vi "MGCC_EnergyMgmt_EMS_HTB.vi"() -> ()   [LabVIEW 2016]
doc: "This VI implements two linear programming models for energy management. The VI uses load and PV forecasting results from the respective functions to generate dispatch of PV and battery for the next 24 hours. Other constraints on the battery and electricity price information are custom inputs and should be specified prior to executing this function."
uses:
  Communication/Global communication.vi
  Communication/Global communication output.vi
  <vilib>/imath/engines/lvmath2/RunTimeEngine/RangeToken/NIMS_Range_R2 - Integer.vi
  <instcachedir>/0/NIMS_Range_R2 - Integer_89B873E74E6E489885E44F751DD9C6BF.lvgen/NIMS_Range_R2 - Integer_89B873E74E6E489885E44F751DD9C6BF_000.vi
  <vilib>/imath/engines/lvmath2/RunTimeEngine/CommandStatement/MC_CommandStatement_break.vi
  <vilib>/imath/engines/lvmath2/RunTimeEngine/VariableToken/NIMS_VariableToken_CondDefinedDefinedByReplace.vi
  <instcachedir>/0/NIMS_VariableToken_CondDefinedDefinedByReplace_D162CFFC24174562A9FEA619A91E1A56.lvgen/NIMS_VariableToken_CondDefinedDefinedByReplace_D162CFFC24174562A9FEA619A91E1A56_004.vi
  <vilib>/imath/engines/lvmath2/RunTimeEngine/IndexRead/NIMS V(R2).vi
  <instcachedir>/0/NIMS V(R2)_C76619605A0E4E9F8B2FA9389712AC47.lvgen/NIMS V(R2)_C76619605A0E4E9F8B2FA9389712AC47_000.vi
  <vilib>/imath/engines/lvmath2/RunTimeEngine/BuiltInFunctions/sum/NIMS_sum(GV).vi
  <instcachedir>/0/NIMS_sum(GV)_67F5EC36BC034E54A6BEC5B0673C00E5.lvgen/NIMS_sum(GV)_67F5EC36BC034E54A6BEC5B0673C00E5_000.vi
  <vilib>/imath/engines/lvmath2/RunTimeEngine/IndexReplace/NIMS V(S)=S.vi
  <instcachedir>/0/NIMS V(S)=S_57E16554CB8B4B90AAB163894F717546.lvgen/NIMS V(S)=S_57E16554CB8B4B90AAB163894F717546_000.vi
  <vilib>/imath/engines/lvmath2/RunTimeEngine/ErrorHandling/NIMS_Create Error From Enums.vi
  <vilib>/imath/engines/lvmath2/RunTimeEngine/VariableToken/NIMS_VariableToken_CondDefined.vi
  <instcachedir>/0/NIMS_VariableToken_CondDefined_06E9DA95BD4D46A6BA55EC651A891960.lvgen/NIMS_VariableToken_CondDefined_06E9DA95BD4D46A6BA55EC651A891960_006.vi
  <vilib>/imathl/engines/lvmath/Functions/Error Handling/Create Error.vi
  <vilib>/imath/engines/lvmath2/RunTimeEngine/BuiltInFunctions/is_nan/NIMS_is_nan.vi
  <instcachedir>/0/NIMS_is_nan_BCCD798162CC49E3A8E57072444F6EB6.lvgen/NIMS_is_nan_BCCD798162CC49E3A8E57072444F6EB6_003.vi
  <vilib>/imath/engines/lvmath2/RunTimeEngine/BuiltInFunctions/max/1 input/NIMS_max(RV).vi
  <instcachedir>/0/NIMS_max(RV)_237633DB1D604D5BA7001287DF3C7957.lvgen/NIMS_max(RV)_237633DB1D604D5BA7001287DF3C7957_002.vi
  <vilib>/imath/engines/lvmath2/RunTimeEngine/BuiltInFunctions/tril/NIMS_tril.vi
  <instcachedir>/0/NIMS_tril_6D22CCA5CB604C1FB8874D0E0A590B2C.lvgen/NIMS_tril_6D22CCA5CB604C1FB8874D0E0A590B2C_003.vi
  <vilib>/imath/engines/lvmath2/RunTimeEngine/RowToken/NIMS_RowToken_M_CV.vi
  <instcachedir>/0/NIMS_RowToken_M_CV_FA79F1D1D17D44459F3ED8E09EE8B625.lvgen/NIMS_RowToken_M_CV_FA79F1D1D17D44459F3ED8E09EE8B625_002.vi
  <vilib>/imath/engines/lvmath2/RunTimeEngine/MatrixToken/NIMS_MatrixToken_M_M.vi
  <instcachedir>/0/NIMS_MatrixToken_M_M_DF273B0CC20F424BBF1EDA9F4E71C841.lvgen/NIMS_MatrixToken_M_M_DF273B0CC20F424BBF1EDA9F4E71C841_005.vi
  <vilib>/imath/engines/lvmath2/RunTimeEngine/ArithmeticOperatorToken/NIMS_ArithmeticOperator_minus.vi
  <instcachedir>/0/NIMS_ArithmeticOperator_minus_E3B65B1D26A44BB184AFDC5B3F458E3D.lvgen/NIMS_ArithmeticOperator_minus_E3B65B1D26A44BB184AFDC5B3F458E3D_003.vi
  <vilib>/imath/engines/lvmath2/RunTimeEngine/BuiltInFunctions/double/NIMS_double.vi
  <instcachedir>/0/NIMS_double_34E32F64C2B04A25A042F4CA881A0A41.lvgen/NIMS_double_34E32F64C2B04A25A042F4CA881A0A41_000.vi
  <instcachedir>/0/NIMS_double_34E32F64C2B04A25A042F4CA881A0A41.lvgen/NIMS_double_34E32F64C2B04A25A042F4CA881A0A41_003.vi
  <instcachedir>/0/NIMS_double_34E32F64C2B04A25A042F4CA881A0A41.lvgen/NIMS_double_34E32F64C2B04A25A042F4CA881A0A41_002.vi
  <vilib>/imath/engines/lvmath2/RunTimeEngine/RowToken/NIMS_RowToken_M_M.vi
  <instcachedir>/0/NIMS_RowToken_M_M_968CDE3545E74ACDAEA4B48DE01EEECA.lvgen/NIMS_RowToken_M_M_968CDE3545E74ACDAEA4B48DE01EEECA_004.vi
  <vilib>/imath/engines/lvmath2/RunTimeEngine/MatrixToken/NIMS_MatrixToken_M_RV.vi
  <instcachedir>/0/NIMS_MatrixToken_M_RV_EE14907D4B194E829889005D2F556E9C.lvgen/NIMS_MatrixToken_M_RV_EE14907D4B194E829889005D2F556E9C_001.vi
  <instcachedir>/0/NIMS_MatrixToken_M_M_DF273B0CC20F424BBF1EDA9F4E71C841.lvgen/NIMS_MatrixToken_M_M_DF273B0CC20F424BBF1EDA9F4E71C841_004.vi
  <vilib>/imath/engines/lvmath/Functions/Error Handling/MergeErrorsWrapper.vi
  <vilib>/imath/engines/lvmath2/RunTimeEngine/BuiltInFunctions/fmin_lp/NIMS_fmin_lp.vi
  <vilib>/imath/engines/lvmath2/RunTimeEngine/IndexRead/NIMS V(S).vi
  <instcachedir>/0/NIMS V(S)_0488751826AF41519A22953C041130DC.lvgen/NIMS V(S)_0488751826AF41519A22953C041130DC_000.vi
  <instcachedir>/0/NIMS_max(RV)_237633DB1D604D5BA7001287DF3C7957.lvgen/NIMS_max(RV)_237633DB1D604D5BA7001287DF3C7957_000.vi
  <vilib>/imath/engines/lvmath2/RunTimeEngine/NodeEndStatement/NIMS_NodeEndStatement_Output.vi
  <instcachedir>/0/NIMS_NodeEndStatement_Output_53EC0D466D134D7ABD903AC30B43404B.lvgen/NIMS_NodeEndStatement_Output_53EC0D466D134D7ABD903AC30B43404B_005.vi
  <instcachedir>/0/NIMS_NodeEndStatement_Output_53EC0D466D134D7ABD903AC30B43404B.lvgen/NIMS_NodeEndStatement_Output_53EC0D466D134D7ABD903AC30B43404B_001.vi
  <instcachedir>/0/NIMS_NodeEndStatement_Output_53EC0D466D134D7ABD903AC30B43404B.lvgen/NIMS_NodeEndStatement_Output_53EC0D466D134D7ABD903AC30B43404B_011.vi
  <vilib>/imath/engines/lvmath2/RunTimeEngine/ErrorHandling/NIMS_Finalize Error.vi
  f_MGCC_EnergyMgmt_CostSavings.vi
  Battery Dispatch.vi
  <instcachedir>/0/NIMS_RowToken_M_M_968CDE3545E74ACDAEA4B48DE01EEECA.lvgen/NIMS_RowToken_M_M_968CDE3545E74ACDAEA4B48DE01EEECA_005.vi
  <vilib>/imath/engines/lvmath2/RunTimeEngine/MatrixToken/NIMS_MatrixToken_M_SorCV.vi
  <instcachedir>/0/NIMS_MatrixToken_M_SorCV_D3266533510A4291A747E91CF193467A.lvgen/NIMS_MatrixToken_M_SorCV_D3266533510A4291A747E91CF193467A_001.vi
  <vilib>/imath/engines/lvmath2/RunTimeEngine/BuiltInFunctions/length/NIMS_length(GV).vi
  <instcachedir>/0/NIMS_length(GV)_08A3D13377FD4E4B96F5795FBF3698FA.lvgen/NIMS_length(GV)_08A3D13377FD4E4B96F5795FBF3698FA_002.vi
  <vilib>/imath/engines/lvmath2/RunTimeEngine/BuiltInFunctions/eye/NIMS_M=eye(I32).vi
  <vilib>/Utility/error.llb/Error Cluster From Error Code.vi
  <vilib>/ErrorRing/Error Ring.xnode
  Lib/MGCC_EnergyMgmt_dataIO.lvlib
panel:
  out "Dispatched loads":dbl[](graph)
  out "Dispatched PV ISD":dbl[](graph)
  out "Forecast PV":dbl[](graph)
  out "Forecast Load":dbl[](graph)
  out "Battery Dispatch":dbl[](graph)
  out "Net load after":dbl[](graph)
  out "Net load b4":dbl[](graph)
  out "Savings":dbl
  out "error out ISD":errorcluster
  out "ISD_EMS_BATT":dbl[](array[numeric])
  out "ISD_EMS_PV":dbl[](array[numeric])
  out "Load_Forecast_GC":dbl[](array[numeric])
  out "P_batt":dbl[](array[numeric])
  out "PV_Forecast_GC":dbl[](array[numeric])
  out "error out GC":errorcluster
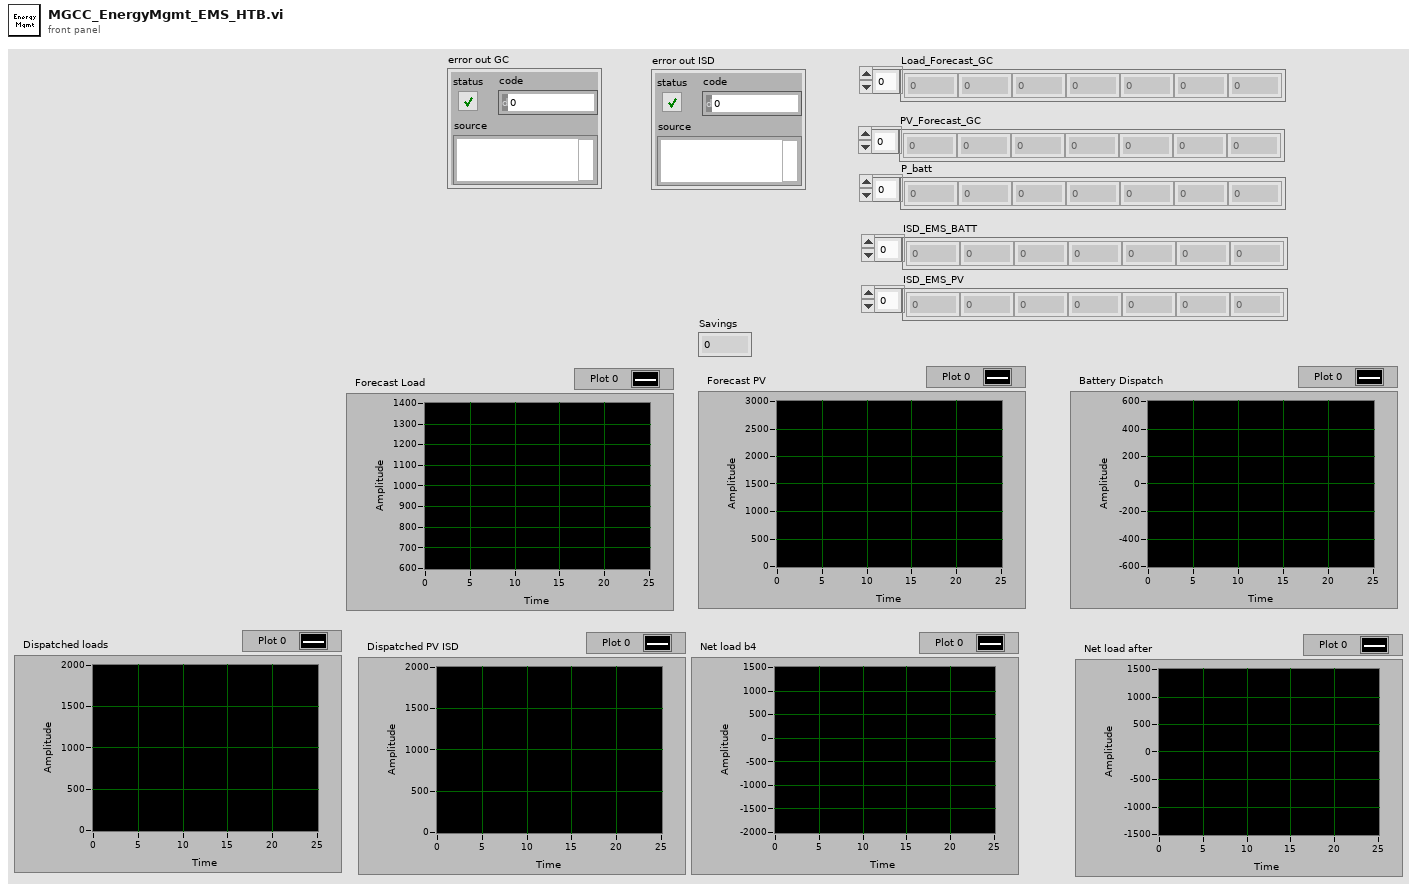
[diagram p1: front panel]
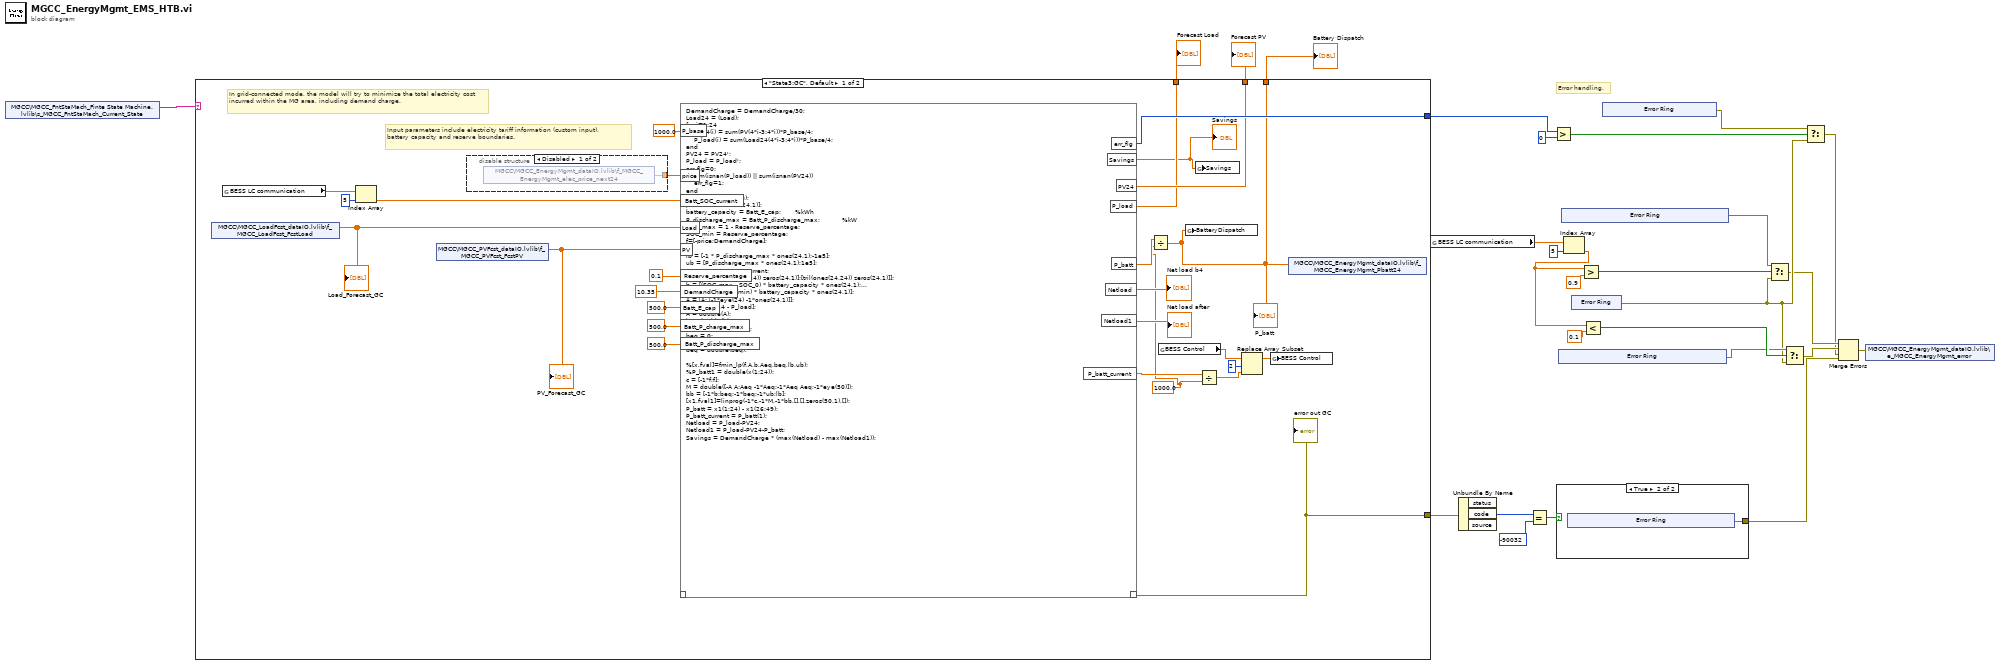
[diagram p0: block diagram]
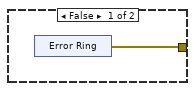
[diagram p2: hidden frame]
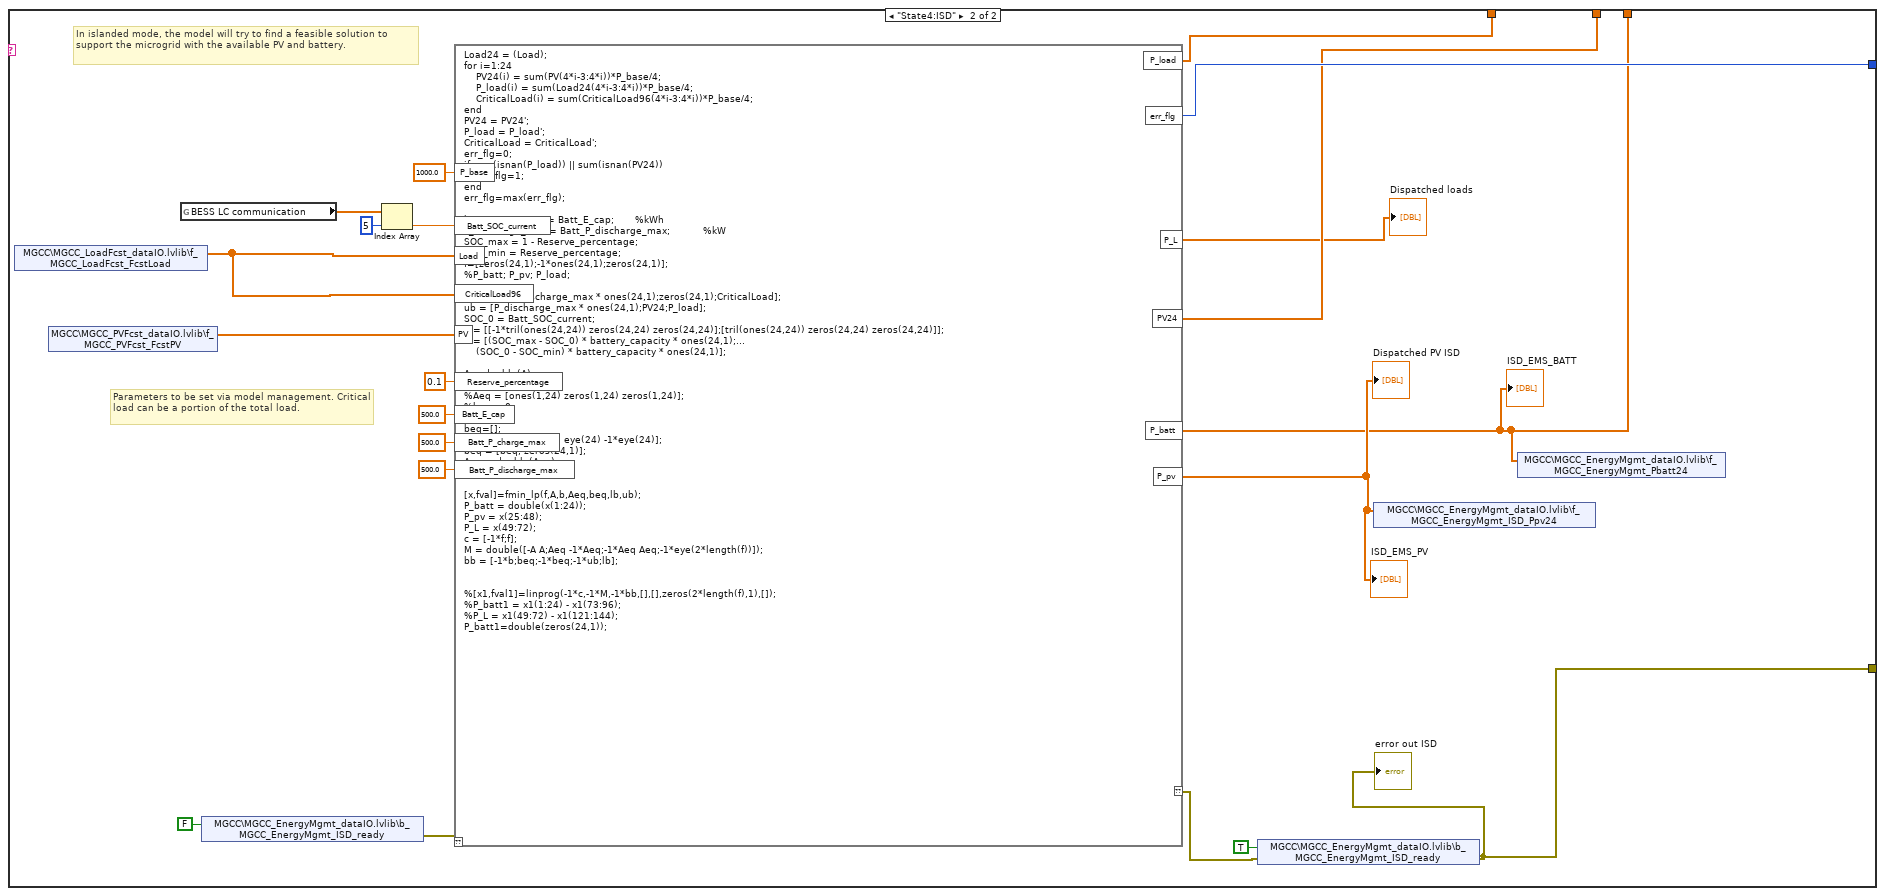
[diagram p4: hidden frame]
diagram:
  # "Error handling."
  n1 = shared-variable "MGCC\\MGCC_FntStaMach_Finte State Machine.lvlib\\s_MGCC_FntStaMach_Current_State"() -> (w27:string)  [unwired: 1 in, 1 out]
  n2 = case shown="\"State3:GC\", Default" w27 {
    tunnel: [w46 w740] -> w19
    tunnel: [w36 w732] -> w5
    tunnel: [w33 w737] -> w8
    tunnel: [w32 w738] -> w7
    tunnel: [w28 w733] -> w6
    frame "State3:GC", Default {
      w29 = 1000.0 ("y")
      # "In grid-connected mode, the model will try to minimize the total electricity cost incurred within the MG area, including demand charge."
      # "Input parameters include electricity tariff information (custom input), battery capacity and reserve boundaries."
      n3 = shared-variable "MGCC\\MGCC_LoadFcst_dataIO.lvlib\\f_MGCC_LoadFcst_FcstLoad"() -> (w45:dbl[])  [unwired: 1 in, 1 out]
      "Load_Forecast_GC" <- w45
      n4 = global read "Global communication.vi" "BESS LC communication"() -> (w44:dbl[])
      n5 = Index Array(array=w44, index=5) -> (element=w42:dbl)
      n6 = shared-variable "MGCC\\MGCC_PVFcst_dataIO.lvlib\\f_MGCC_PVFcst_FcstPV"() -> (w49:dbl[])  [unwired: 1 in, 1 out]
      "PV_Forecast_GC" <- w49
      n7 = disable-structure shown="Disabled" {
        disable-tunnel: [w55 _] -> w54
        frame Disabled {
          n8 = shared-variable "MGCC\\MGCC_EnergyMgmt_dataIO.lvlib\\f_MGCC_EnergyMgmt_elec_price_next24"() -> (w55:dbl[])  [unwired: 1 in, 1 out]
        }
        frame Enabled {
        }
      }
      n9 = mathscript code="DemandCharge = DemandCharge/30;\nLoad24 = (Load);\nfor i=1:24\n    PV24(i) = sum(PV(4*i-3:4*i))*P_base/4;\n    P_load(i) = sum(Load24(4*i-3:4*i))*P_base/4;\nend\nPV24 = PV24';\nP_load = P_load';\nerr_flg=0;\nif sum(isnan(P_load)) || sum(isnan(PV24))\n    err_flg=1;\nend\nerr_flg=max(err_flg);\nprice=[0.06*ones(24,1)];\nbattery_capacity = Batt_E_cap;       %kWh\nP_discharge_max = Batt_P_discharge_max;           %kW\nSOC_max = 1 - Reserve_percentage;\nSOC_min = Reserve_percentage;\nf=[-price;DemandCharge];\n\nlb = [-1 * P_discharge_max * ones(24,1);-1e5];\nub = [P_discharge_max * ones(24,1);1e5];\nSOC_0 = Batt_SOC_current;\nA = [[-1*tril(ones(24,24)) zeros(24,1)];[tril(ones(24,24)) zeros(24,1)]];\nb = [(SOC_max - SOC_0) * battery_capacity * ones(24,1);...\n    (SOC_0 - SOC_min) * battery_capacity * ones(24,1)];\nA = [A; [-1*eye(24) -1*ones(24,1)]];\nb = [b; PV24 - P_load];\nA = double(A);\nb = double(b);\nAeq = [ones(1,24) 0];\nbeq = 0;\nAeq = double(Aeq);\nbeq = double(beq);\n\n%[x,fval]=fmin_lp(f,A,b,Aeq,beq,lb,ub);\n%P_batt1 = double(x(1:24));\nc = [-1*f;f];\nM = double([-A A;Aeq -1*Aeq;-1*Aeq Aeq;-1*eye(50)]);\nbb = [-1*b;beq;-1*beq;-1*ub;lb];\n[x1,fval1]=linprog(-1*c,-1*M,-1*bb,[],[],zeros(50,1),[]);\nP_batt = x1(1:24) - x1(26:49);\nP_batt_current = P_batt(1);\nNetload = P_load-PV24;\nNetload1 = P_load-PV24-P_batt;\nSavings = DemandCharge * (max(Netload) - max(Netload1));"("price"=w54, "Batt_E_cap"=500.0, "Batt_P_charge_max"=500.0, "Batt_P_discharge_max"=500.0, "Batt_SOC_current"=w42, "DemandCharge"=10.35, "Load"=w45, "PV"=w49, "Reserve_percentage"=0.1, "P_base"=1000.0) -> ("??"=w36:errorcluster, "P_batt"=w30:dbl[], "P_batt_current"=w47:dbl, "err_flg"=w46:i32, "Savings"=w31:dbl, "PV24"=w33:dbl[], "P_load"=w32:dbl[], "Netload"=→"Net load b4":dbl[], "Netload1"=→"Net load after":dbl[])  [unwired: 1 in]
      "error out GC" <- w36
      "Savings" <- w31
      n10 = Divide(x=w30, y=w29) -> (x/y=w28:dbl[])
      "P_batt" <- w28
      n11 = global read "Global communication output.vi" "BESS Control"() -> (w41:dbl[])
      n12 = global write "Battery Dispatch.vi" "BatteryDispatch"(w28) -> ()
      n13 = global write "f_MGCC_EnergyMgmt_CostSavings.vi" "Savings"(w31) -> ()
      n14 = Divide(x=w47, y=w29) -> (x/y=w39:dbl)
      n15 = Replace Array Subset(array=w41, new element=w39, index=2) -> (w38:dbl[])
      n16 = global write "Global communication output.vi" "BESS Control"(w38) -> ()
      n17 = shared-variable "MGCC\\MGCC_EnergyMgmt_dataIO.lvlib\\f_MGCC_EnergyMgmt_Pbatt24"(w28) -> ()  [unwired: 1 in, 1 out]
    }
    frame "State4:ISD" {
      # "In islanded mode, the model will try to find a feasible solution to support the microgrid with the available PV and battery."
      # "Parameters to be set via model management. Critical load can be a portion of the total load."
      n18 = shared-variable "MGCC\\MGCC_LoadFcst_dataIO.lvlib\\f_MGCC_LoadFcst_FcstLoad"() -> (w736:dbl[])  [unwired: 1 in, 1 out]
      n19 = shared-variable "MGCC\\MGCC_PVFcst_dataIO.lvlib\\f_MGCC_PVFcst_FcstPV"() -> (w745:dbl[])  [unwired: 1 in, 1 out]
      n20 = global read "Global communication.vi" "BESS LC communication"() -> (w750:dbl[])
      n21 = shared-variable "MGCC\\MGCC_EnergyMgmt_dataIO.lvlib\\b_MGCC_EnergyMgmt_ISD_ready"(FALSE ("b_MGCC_EnergyMgmt_ISD_ready")) -> (error out=w746:errorcluster)  [unwired: 1 in]
      n22 = Index Array(array=w750, index=5) -> (element=w748:dbl)
      n23 = mathscript code="Load24 = (Load);\nfor i=1:24\n    PV24(i) = sum(PV(4*i-3:4*i))*P_base/4;\n    P_load(i) = sum(Load24(4*i-3:4*i))*P_base/4;\n    CriticalLoad(i) = sum(CriticalLoad96(4*i-3:4*i))*P_base/4;\nend\nPV24 = PV24';\nP_load = P_load';\nCriticalLoad = CriticalLoad';\nerr_flg=0;\nif sum(isnan(P_load)) || sum(isnan(PV24))\n    err_flg=1;\nend\nerr_flg=max(err_flg);\n\nbattery_capacity = Batt_E_cap;       %kWh\nP_discharge_max = Batt_P_discharge_max;           %kW\nSOC_max = 1 - Reserve_percentage;\nSOC_min = Reserve_percentage;\nf=[zeros(24,1);-1*ones(24,1);zeros(24,1)];\n%P_batt; P_pv; P_load;\n\nlb = [-1 * P_discharge_max * ones(24,1);zeros(24,1);CriticalLoad];\nub = [P_discharge_max * ones(24,1);PV24;P_load];\nSOC_0 = Batt_SOC_current;\nA = [[-1*tril(ones(24,24)) zeros(24,24) zeros(24,24)];[tril(ones(24,24)) zeros(24,24) zeros(24,24)]];\nb = [(SOC_max - SOC_0) * battery_capacity * ones(24,1);...\n    (SOC_0 - SOC_min) * battery_capacity * ones(24,1)];\n\nA = double(A);\nb = double(b);\n%Aeq = [ones(1,24) zeros(1,24) zeros(1,24)];\n%beq = 0;\nAeq=[];\nbeq=[];\nAeq = [Aeq; eye(24) eye(24) -1*eye(24)];\nbeq = [beq; zeros(24,1)];\nAeq = double(Aeq);\nbeq = double(beq);\n\n[x,fval]=fmin_lp(f,A,b,Aeq,beq,lb,ub);\nP_batt = double(x(1:24));\nP_pv = x(25:48);\nP_L = x(49:72);\nc = [-1*f;f];\nM = double([-A A;Aeq -1*Aeq;-1*Aeq Aeq;-1*eye(2*length(f))]);\nbb = [-1*b;beq;-1*beq;-1*ub;lb];\n\n\n%[x1,fval1]=linprog(-1*c,-1*M,-1*bb,[],[],zeros(2*length(f),1),[]);\n%P_batt1 = x1(1:24) - x1(73:96);\n%P_L = x1(49:72) - x1(121:144);\nP_batt1=double(zeros(24,1));"("??"=w746, "Batt_E_cap"=500.0, "Batt_P_charge_max"=500.0, "Batt_P_discharge_max"=500.0, "Batt_SOC_current"=w748, "Load"=w736, "PV"=w745, "Reserve_percentage"=0.1, "CriticalLoad96"=w736, "P_base"=1000.0) -> ("??"=w731:errorcluster, "P_L"=→"Dispatched loads":dbl[], "err_flg"=w740:i32, "PV24"=w737:dbl[], "P_load"=w738:dbl[], "P_batt"=w733:dbl[], "P_pv"=w734:dbl[])
      "ISD_EMS_PV" <- w734
      "ISD_EMS_BATT" <- w733
      "Dispatched PV ISD" <- w734
      n24 = shared-variable "MGCC\\MGCC_EnergyMgmt_dataIO.lvlib\\b_MGCC_EnergyMgmt_ISD_ready"(TRUE ("b_MGCC_EnergyMgmt_ISD_ready"), error in=w731) -> (error out=w732:errorcluster)
      "error out ISD" <- w732
      n25 = shared-variable "MGCC\\MGCC_EnergyMgmt_dataIO.lvlib\\f_MGCC_EnergyMgmt_ISD_Ppv24"(w734) -> ()  [unwired: 1 in, 1 out]
      n26 = shared-variable "MGCC\\MGCC_EnergyMgmt_dataIO.lvlib\\f_MGCC_EnergyMgmt_Pbatt24"(w733) -> ()  [unwired: 1 in, 1 out]
    }
  }
  "Forecast Load" <- w7
  "Forecast PV" <- w8
  "Battery Dispatch" <- w6
  n27 = global read "Global communication.vi" "BESS LC communication"() -> (w11:dbl[])
  n28 = Unbundle By Name(w5) -> ("code"=w4:i32)  [unwired: 2 out]
  n29 = Equal?(x=w4, y=-90032) -> (x = y?=w2:bool)
  n30 = Greater?(x=w19, y=0) -> (0:w18:bool)
  n31 = case shown="True" w2 {
    tunnel: [w1453 w1455] -> w1
    frame False {
      n32 = xnode "Error Ring"() -> ("error out"=w1453:errorcluster)
    }
    frame True {
      n33 = xnode "Error Ring"() -> ("error out"=w1455:errorcluster)
    }
  }
  n34 = xnode "Error Ring"() -> ("error out"=w21:errorcluster)
  n35 = xnode "Error Ring"() -> ("error out"=w23:errorcluster)
  n36 = Index Array(array=w11, index=5) -> (element=w9:dbl)
  n37 = xnode "Error Ring"() -> ("error out"=w16:errorcluster)
  n38 = Greater?(x=w9, y=0.9) -> (0:w24:bool)
  n39 = Less?(x=w9, y=0.1) -> (x < y?=w22:bool)
  n40 = xnode "Error Ring"() -> ("error out"=w17:errorcluster)
  n41 = Select(t=w23, s=w24, f=w16) -> (s? t:f=w15:errorcluster)
  n42 = Select(t=w21, s=w22, f=w16) -> (s? t:f=w14:errorcluster)
  n43 = Select(t=w17, s=w18, f=w16) -> (s? t:f=w13:errorcluster)
  n44 = Merge Errors(w15, w14, w13, w1) -> (w12:errorcluster)
  n45 = shared-variable "MGCC\\MGCC_EnergyMgmt_dataIO.lvlib\\e_MGCC_EnergyMgmt_error"(w12) -> ()  [unwired: 1 in, 1 out]
